vi "Admin Enable Globalv2.vi"() -> ()   [LabVIEW 2014, in "Main Libraryv2.lvlib"]
uses:
  Control/Main Libraryv2.lvlib
panel:
  out "Admin Enable":bool
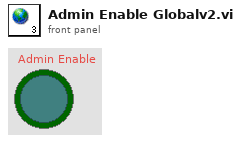
[diagram p1: front panel]
diagram:
